vi "Rename TTL.vi"(8 "error in (no error)":errorcluster, 9 "New name":string, 10 "Old name":string, 11 "Tosca in":refnum<class "Parameters.lvclass">) -> (0 "error out":errorcluster, 3 "Tosca out":refnum<class "Parameters.lvclass">)   [LabVIEW 2015, in "Parameters.lvclass"]
uses:
  Parameters.lvclass
  Parameters.lvclass/Parameters.ctl
  State/State.lvclass
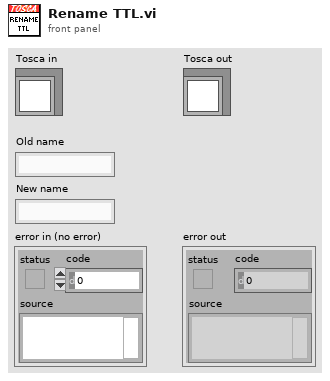
[diagram p1: front panel]
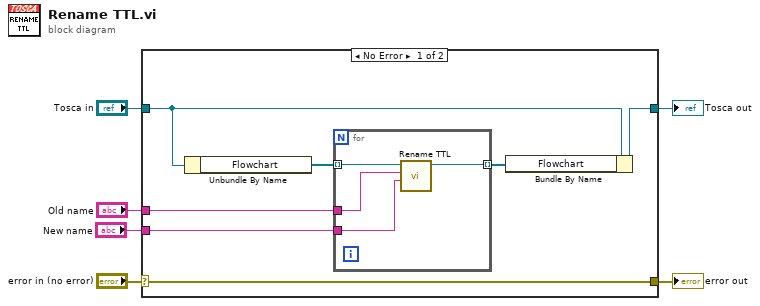
[diagram p0: block diagram]
diagram:
  n1 = case shown="No Error" "error in (no error)" {
    selector: "error in (no error)" -> [w13 w19]
    tunnel: [w13 w19] -> w5
    tunnel: [w10 w18] -> w3
    tunnel: "Tosca in" -> [w12 w18]
    tunnel: "Old name" -> [w8 _]
    tunnel: "New name" -> [w7 _]
    frame No Error {
      n2 = Unbundle By Name(w12) -> ("Flowchart"=w11:refnum<class "State.lvclass">[])
      n3 = for {
        tunnel: w11 -> [w17] mode=indexing
        tunnel: [w14] -> w9 mode=indexing
        tunnel: w8 -> [w16]
        tunnel: w7 -> [w15]
        n4 = call "Rename TTL.vi"("New Name"=w15, "Old Name"=w16, "State in"=w17) -> ("State out"=w14:refnum<class "State.lvclass">)  [unwired: 7 in, 1 out]
      }
      n5 = Bundle By Name(cluster=w12, "Flowchart"=w9) -> (w10:refnum<class "Parameters.lvclass">)
    }
    frame Error {
    }
  }
  "error out" <- w5
  "Tosca out" <- w3
